vi "APS set servo on.vi"(8 "error in (no error)":errorcluster caption="错误输入（无错误）", 10 "Servo_On":i32, 11 "Axis_ID":i32) -> (0 "error out":errorcluster caption="错误输出", 2 "Axis_ID 2":i32, 3 "function return":i32)   [LabVIEW 2017]
doc: "I32 FNTYPE APS_set_servo_on( I32 Axis_ID, I32 Servo_On );"
uses:
  APS168.dll
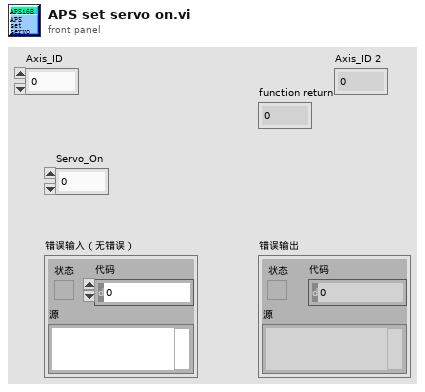
[diagram p1: front panel]
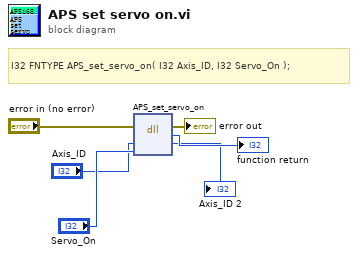
[diagram p0: block diagram]
diagram:
  # "I32 FNTYPE APS_set_servo_on( I32 Axis_ID, I32 Servo_On );"
  n1 = dll-call lib="PTH2Labs E迈治LV范例testSubVIsADLINKLLB运动204cAPS168.*" fn="APS_set_servo_on"(error in="error in (no error)", "Axis_ID"="Axis_ID", "Servo_On"="Servo_On") -> (error out=→"error out":errorcluster, "return type"=→"function return":i32, "Axis_ID"=→"Axis_ID 2":i32)  [unwired: 3 in, 1 out]
